vi "BNO055 read v.2.vi"(8 "error in (no error)":errorcluster, 11 "I2C in":refnum<class "I2C.lvclass">) -> (0 "error out":errorcluster, 1 "pitch":dbl, 2 "roll":dbl, 3 "I2C out":refnum<class "I2C.lvclass">, 4 "yaw":dbl)   [LabVIEW 2019]
uses:
  FPGA_subVIs/low level/I2C/I2C.lvclass
panel:
  in  "Timeout ms (1000)":i32=2
  out "Bytes Read":u8[](array[numeric])
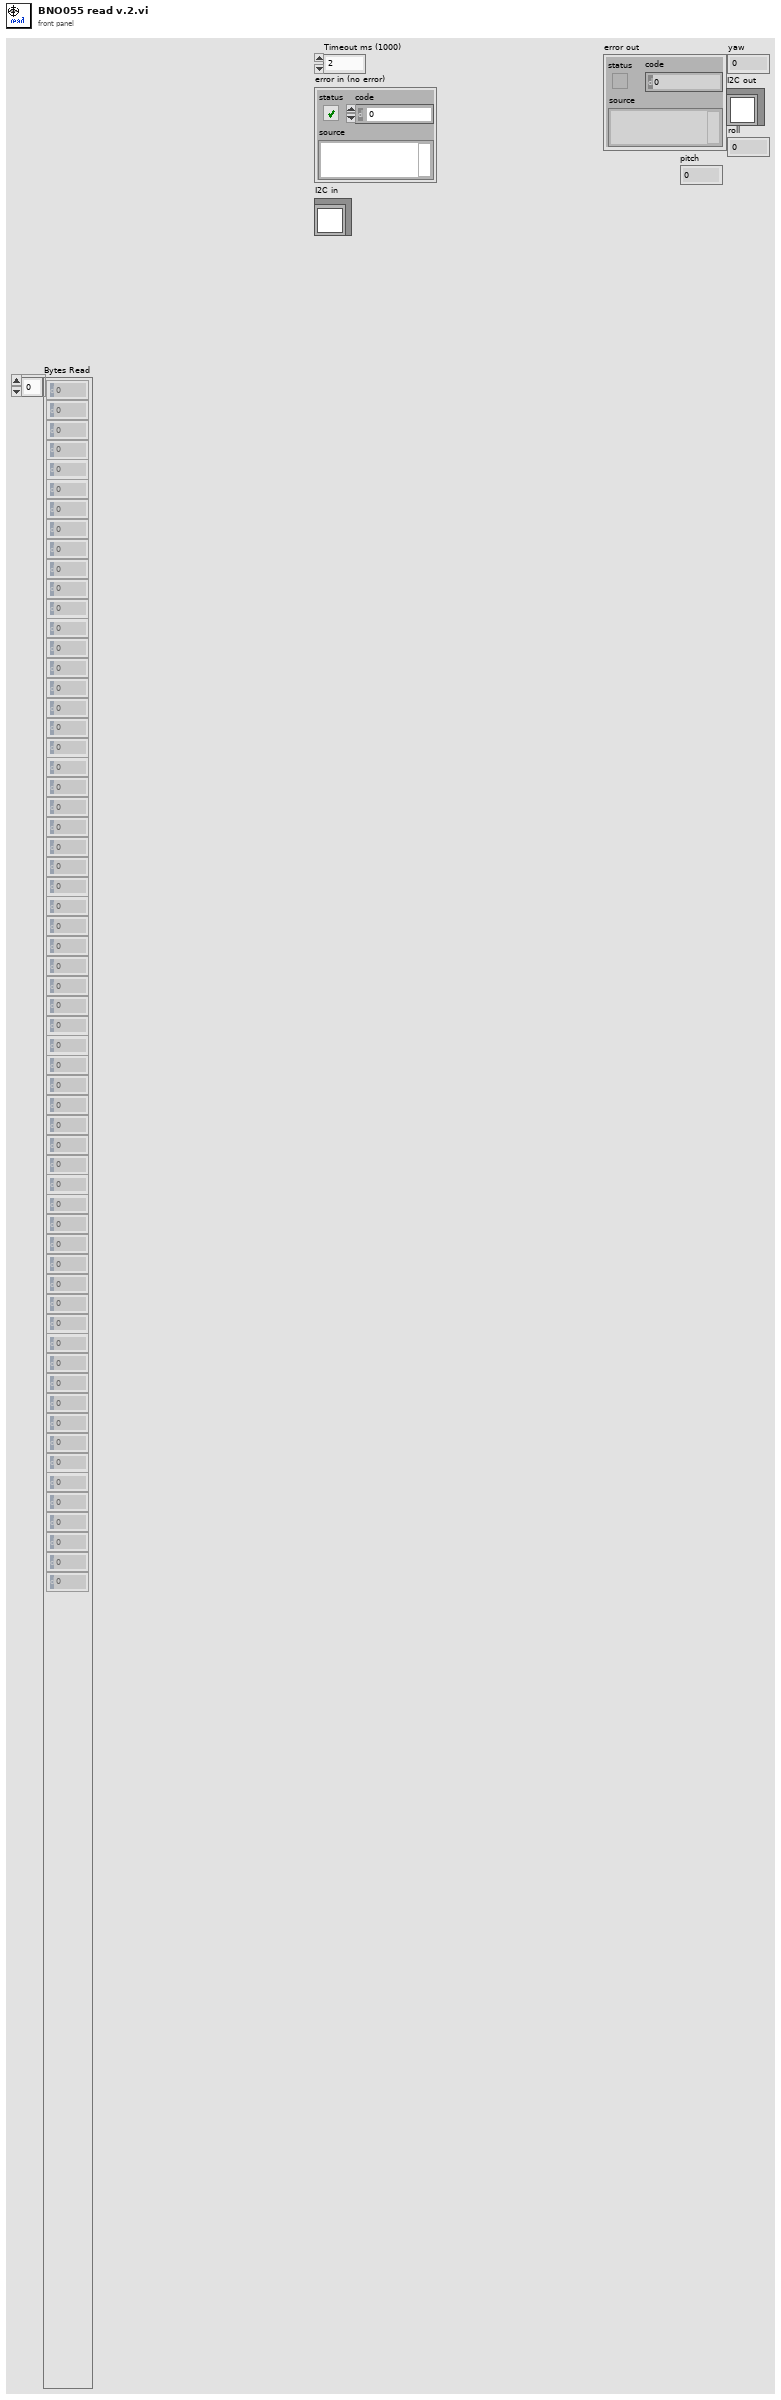
[diagram p1: front panel]
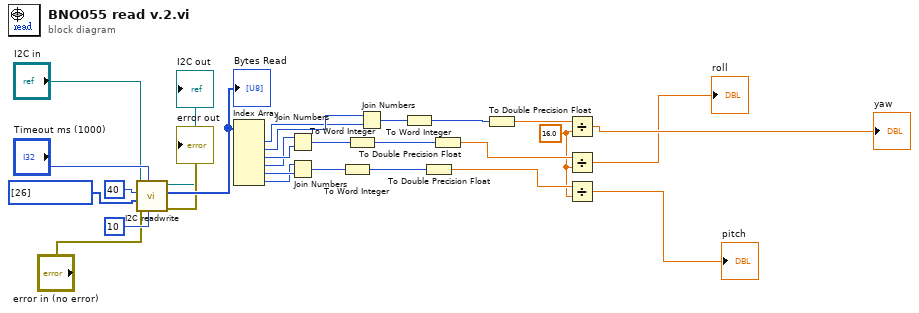
[diagram p0: block diagram]
diagram:
  w6 = 16.0 ("y")
  n1 = call-dynamic "I2C readwrite.vi"("Byte Count"=u32 10, "Timeout ms (1000)"="Timeout ms (1000)", "error in (no error)"="error in (no error)", "Bytes to Write"=u8[] [26], "Slave Address (7-bit)"=u8 40, "I2C in"="I2C in") -> ("error out"=→"error out":errorcluster, "Bytes Read"=w25:u8[], "I2C out"=→"I2C out":refnum<class "I2C.lvclass">)  [unwired: 3 in]
  "Bytes Read" <- w25
  n2 = Index Array(array=w25) -> (element #1=w19:u8, element #2=w22:u8, element #3=w24:u8, element #4=w21:u8, element #5=w23:u8, element #6=w20:u8)  [unwired: 6 in]
  n3 = Join Numbers(hi=w21, lo=w24) -> ((hi.lo)=w10:u16)
  n4 = Join Numbers(hi=w20, lo=w23) -> ((hi.lo)=w9:u16)
  n5 = To Word Integer(number=w9) -> (16bit integer=w3:i16)
  n6 = To Word Integer(number=w10) -> (16bit integer=w2:i16)
  n7 = Join Numbers(hi=w22, lo=w19) -> ((hi.lo)=w18:u16)
  n8 = To Word Integer(number=w18) -> (16bit integer=w1:i16)
  n9 = To Double Precision Float(number=w3) -> (double precision float=w8:dbl)
  n10 = To Double Precision Float(number=w2) -> (double precision float=w7:dbl)
  n11 = To Double Precision Float(number=w1) -> (double precision float=w17:dbl)
  n12 = Divide(x=w17, y=w6) -> (x/y=→"yaw":dbl)
  n13 = Divide(x=w7, y=w6) -> (x/y=→"roll":dbl)
  n14 = Divide(x=w8, y=w6) -> (x/y=→"pitch":dbl)
